vi "Read current.vi"(8 "error in (no error)":errorcluster, 11 "Product-B in":refnum<class "Product-B.lvclass">) -> (0 "error out":errorcluster, 2 "current":dbl, 3 "Product-B out":refnum<class "Product-B.lvclass">)   [LabVIEW 2018, in "Product-B.lvclass"]
uses:
  Product-B.lvclass
  Product-B.lvclass/Product-B.ctl
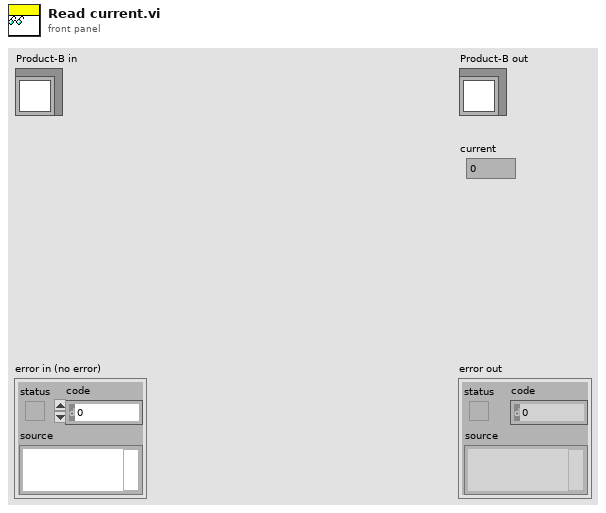
[diagram p1: front panel]
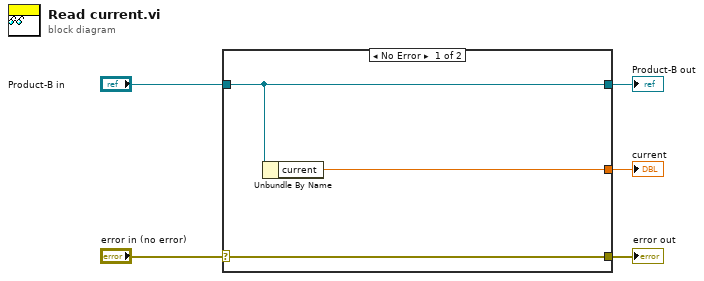
[diagram p0: block diagram]
diagram:
  n1 = case shown="No Error" "error in (no error)" {
    selector: "error in (no error)" -> [w8 w9]
    tunnel: [w8 w9] -> w4
    tunnel: [w7 w10] -> w2
    tunnel: "Product-B in" -> [w7 w10]
    tunnel: [w6 _] -> w1
    frame No Error {
      n2 = Unbundle By Name(w7) -> ("current"=w6:dbl)
    }
    frame Error {
    }
  }
  "error out" <- w4
  "Product-B out" <- w2
  "current" <- w1
